vi "清空文件夹.vi"   [LabVIEW 2018]
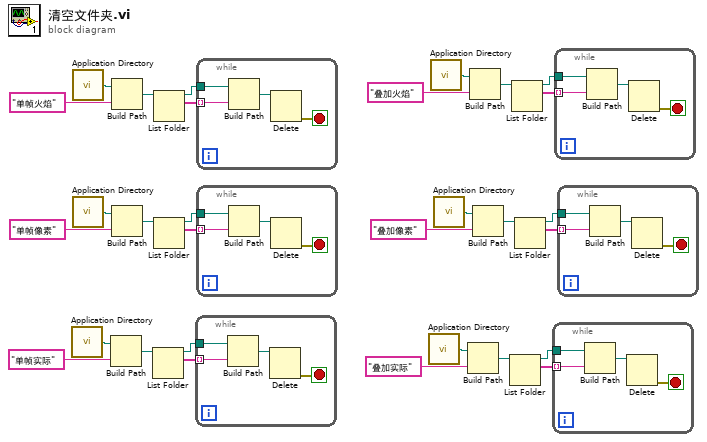
[diagram p0: block diagram]
diagram:
  n1 = call <vilib>:"Application Directory.vi"() -> ("Application Directory"=w17:path)
  n2 = call <vilib>:"Application Directory.vi"() -> ("Application Directory"=w29:path)
  n3 = call <vilib>:"Application Directory.vi"() -> ("Application Directory"=w24:path)
  n4 = Build Path(base path=w17, name or relative path="单帧实际" ("名称或相对路径")) -> (appended path=w19:path)
  n5 = Build Path(base path=w29, name or relative path="单帧火焰" ("名称或相对路径")) -> (appended path=w27:path)
  n6 = Build Path(base path=w24, name or relative path="单帧像素" ("名称或相对路径")) -> (appended path=w22:path)
  n7 = List Folder(path=w19) -> (path out=w16:path, filenames=w20:string[])  [unwired: 3 in, 2 out]
  n8 = List Folder(path=w27) -> (path out=w30:path, filenames=w26:string[])  [unwired: 3 in, 2 out]
  n9 = List Folder(path=w22) -> (path out=w25:path, filenames=w21:string[])  [unwired: 3 in, 2 out]
  n10 = while {
    tunnel: w16 -> [w32]
    tunnel: w20 -> [w31] mode=indexing
    stop <- w34 stop-if-true
    n11 = Build Path(base path=w32, name or relative path=w31) -> (appended path=w33:path)
    n12 = Delete(path (use dialog)=w33) -> (error out=w34:errorcluster)  [unwired: 4 in, 2 out]
  }
  n13 = while {
    tunnel: w30 -> [w36]
    tunnel: w26 -> [w35] mode=indexing
    stop <- w38 stop-if-true
    n14 = Build Path(base path=w36, name or relative path=w35) -> (appended path=w37:path)
    n15 = Delete(path (use dialog)=w37) -> (error out=w38:errorcluster)  [unwired: 4 in, 2 out]
  }
  n16 = while {
    tunnel: w25 -> [w40]
    tunnel: w21 -> [w39] mode=indexing
    stop <- w42 stop-if-true
    n17 = Build Path(base path=w40, name or relative path=w39) -> (appended path=w41:path)
    n18 = Delete(path (use dialog)=w41) -> (error out=w42:errorcluster)  [unwired: 4 in, 2 out]
  }
  n19 = call <vilib>:"Application Directory.vi"() -> ("Application Directory"=w4:path)
  n20 = call <vilib>:"Application Directory.vi"() -> ("Application Directory"=w14:path)
  n21 = call <vilib>:"Application Directory.vi"() -> ("Application Directory"=w7:path)
  n22 = Build Path(base path=w4, name or relative path="叠加实际" ("名称或相对路径")) -> (appended path=w2:path)
  n23 = Build Path(base path=w14, name or relative path="叠加火焰" ("名称或相对路径")) -> (appended path=w12:path)
  n24 = Build Path(base path=w7, name or relative path="叠加像素" ("名称或相对路径")) -> (appended path=w9:path)
  n25 = List Folder(path=w2) -> (path out=w5:path, filenames=w1:string[])  [unwired: 3 in, 2 out]
  n26 = List Folder(path=w12) -> (path out=w15:path, filenames=w11:string[])  [unwired: 3 in, 2 out]
  n27 = List Folder(path=w9) -> (path out=w6:path, filenames=w10:string[])  [unwired: 3 in, 2 out]
  n28 = while {
    tunnel: w5 -> [w44]
    tunnel: w1 -> [w43] mode=indexing
    stop <- w46 stop-if-true
    n29 = Build Path(base path=w44, name or relative path=w43) -> (appended path=w45:path)
    n30 = Delete(path (use dialog)=w45) -> (error out=w46:errorcluster)  [unwired: 4 in, 2 out]
  }
  n31 = while {
    tunnel: w15 -> [w48]
    tunnel: w11 -> [w47] mode=indexing
    stop <- w50 stop-if-true
    n32 = Build Path(base path=w48, name or relative path=w47) -> (appended path=w49:path)
    n33 = Delete(path (use dialog)=w49) -> (error out=w50:errorcluster)  [unwired: 4 in, 2 out]
  }
  n34 = while {
    tunnel: w6 -> [w52]
    tunnel: w10 -> [w51] mode=indexing
    stop <- w54 stop-if-true
    n35 = Build Path(base path=w52, name or relative path=w51) -> (appended path=w53:path)
    n36 = Delete(path (use dialog)=w53) -> (error out=w54:errorcluster)  [unwired: 4 in, 2 out]
  }
